vi "Run Test and Get Suite Result.vi"(8 "error in (no error)":errorcluster, 11 "Test Test Case in":refnum<class "LUnit Test Case.lvclass">) -> (0 "error out":errorcluster, 3 "Test Suite Result out":T1)   [LabVIEW 2020, in "LUnit Tests.lvlib" / "Test Suite Result Test.lvclass"]
uses:
  Test Suite Result Test.lvclass
  source/Framework/Test Case/LUnit Test Case.lvclass
  source/Framework/Result Types/Suite Results/Test Suite Result type.ctl
  source/Framework/Result Types/Assertion Result/Public/TypeDefs/Status.ctl
  source/Framework/Result Types/Case Result/Test Case Result type.ctl
  source/Framework/Result Types/Method Result/Method Result type.ctl
  source/Framework/Result Types/Assertion Result/Assertion Result type.ctl
  source/Framework/Result Types/Assertion Result/Public/TypeDefs/Assertion Type.ctl
  source/Framework/Execution API/Execution API.lvclass
  source/Framework/Result Types/Assertion Result/Assertion Result.lvlib
  source/Framework/Result Types/Method Result/Method Result.lvlib
  source/Framework/Result Types/Case Result/Test Case Result.lvlib
  source/Framework/Result Types/Suite Results/Test Suite Result.lvlib
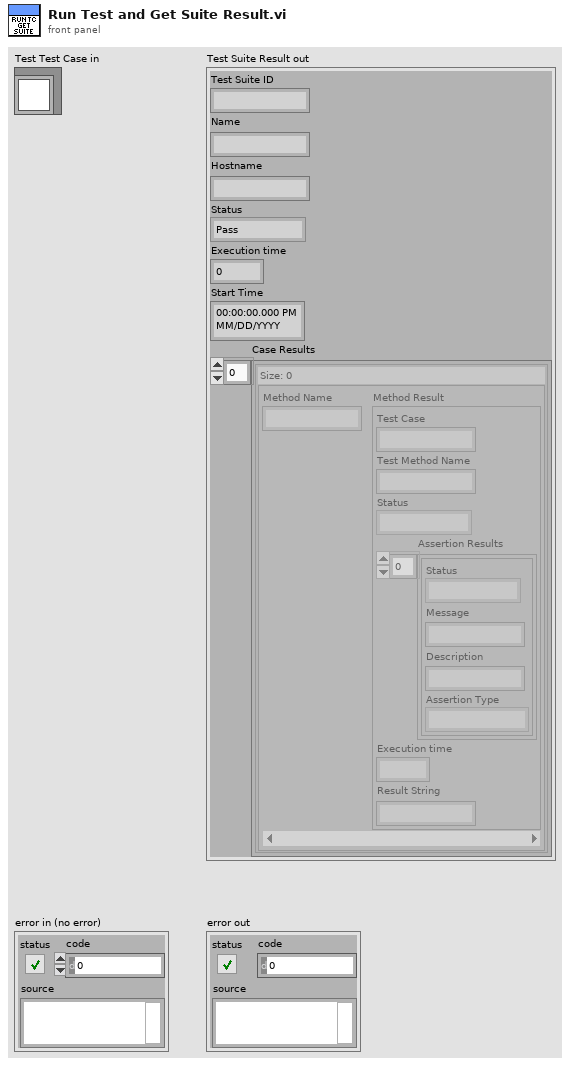
[diagram p1: front panel]
types:
  T1 = typedef "Test Suite Result.lvlib/Test Suite Result type.ctl" = cluster{"Test Suite ID":string, "Name":string, "Hostname":string, "Status":T2, "Execution time":dbl, "Start Time":timestamp, "Case Results":T3[]}
  T2 = typedef "Assertion Result.lvlib/Status.ctl" = enum16{"Pass", "Fail", "Error", "Skipped", "Setup Error", "Broken", "Teardown Error"}
  T3 = typedef "Test Case Result.lvlib/Test Case Result type.ctl" = map{string, T4}
  T4 = typedef "Method Result.lvlib/Method Result type.ctl" = cluster{"Test Case":string, "Test Method Name":string, "Status":T2, "Assertion Results":T5[], "Execution time":dbl, "Result String":string}
  T5 = typedef "Assertion Result.lvlib/Assertion Result type.ctl" = cluster{"Status":T2, "Message":string, "Description":string, "Assertion Type":T6}
  T6 = typedef "Assertion Result.lvlib/Assertion Type.ctl" = enum16{"None", "Pass", "Fail", "Skip", "Pass if Equal", "Fail if Equal", "Pass if Error", "Fail if Error", "Pass if", "Fail if"}
  T7 = cluster{"Result Events":refnum<event-registration>, "Event Registration Refnum":refnum<event-registration>}
  T8 = typedef "Test Case Result.lvlib/Test Case Result.ctl" = map{string, T9}
  T9 = typedef "Method Result.lvlib/Method Result.ctl" = cluster{"Test Case":string, "Test Method Name":string, "Status":T2, "Assertion Results":T10[], "Execution time":dbl, "Result String":string}
  T10 = typedef "Assertion Result.lvlib/Assertion Result.ctl" = cluster{"Status":T2, "Message":string, "Description":string, "Assertion Type":T6}
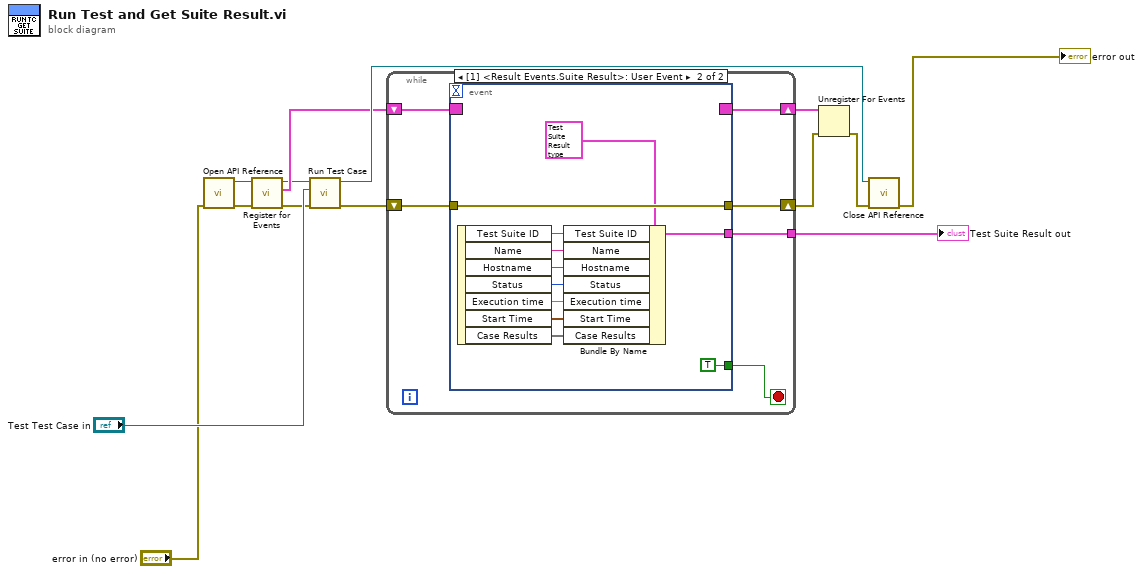
[diagram p0: block diagram]
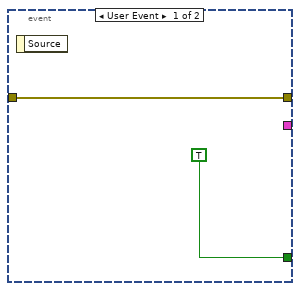
[diagram p2: hidden frame]
diagram:
  n1 = call "Open API Reference.vi"("error in (no error)"="error in (no error)") -> ("error out"=w2:errorcluster, "Execution API out"=w1:refnum<class "Execution API.lvclass">)  [unwired: 9 in]
  n2 = call "Register for Events.vi"("error in (no error)"=w2, "Execution API In"=w1) -> ("error out"=w4:errorcluster, "Result Registration Refnum"=w5:T7, "Execution API Out"=w3:refnum<class "Execution API.lvclass">)  [unwired: 7 in]
  n3 = call "Run Test Case.vi"("error in (no error)"=w4, "Test Case"="Test Test Case in", "Execution API In"=w3) -> ("error out"=w7:errorcluster, "Execution API Out"=w10:refnum<class "Execution API.lvclass">)  [unwired: 7 in]
  n4 = while {
    shift-right: [w19] -> w6
    shift-left: w5 -> [w20]
    shift-right: [w17] -> w8
    shift-left: w7 -> [w18]
    tunnel: [w15] -> w12
    stop <- w16 stop-if-true
    n5 = event shown="[1] <Result Events.Suite Result>: User Event" {
      selector: w20 -> [_ _]
      dyn-events: [_ _] -> w19
      timeout: _ -> [_ _]
      tunnel: w18 -> [w22 w33]
      tunnel: [w22 w33] -> w17
      tunnel: [TRUE TRUE] -> w16
      tunnel: [_ w30] -> w15
      event User Event {
        n6 = event-data() -> ()  [unwired: 1 in, 1 out]
      }
      event User Event {
        n7 = event-data() -> ("Test Suite ID"=w31:string, "Name"=w28:string, "Hostname"=w27:string, "Status"=w26:T2, "Execution time"=w25:dbl, "Start Time"=w24:timestamp, "Case Results"=w23:T8[])  [unwired: 1 in]
        n8 = Bundle By Name(cluster=T1 {"Test Suite ID"="", "Name"="", "Hostname"="", "Status"=enum."Pass", "Execution time"=0.0, "Start Time"=timestamp(0 s since 1904-01-01), "Case Results"=[]} ("Test Suite Result out"), "Test Suite ID"=w31, "Name"=w28, "Hostname"=w27, "Status"=w26, "Execution time"=w25, "Start Time"=w24, "Case Results"=w23) -> (w30:T1)
      }
    }
  }
  "Test Suite Result out" <- w12
  n9 = Unregister For Events(event registration refnum=w6, error in=w8) -> (error out=w9:errorcluster)
  n10 = call "Close API Reference.vi"("error in (no error)"=w9, "Execution API in"=w10) -> ("error out"=→"error out":errorcluster)  [unwired: 9 in]
